vi "Set plot visibility.vi"(9 "Data In":T2, 10 "Timeline":T1, 11 "WaveformGraph in":T7) -> (3 "WaveformGraph out":T7)   [LabVIEW 2017, in "XGrapher.xctl"]
uses:
  XGrapher.xctl
  Typedefs/Xctrl-Waveform graph ref.ctl
  Data 1.ctl
  Typedefs/Xctrl-Data array.ctl
  Typedefs/Xcrtl-Data format definition.ctl
  Typedefs/Xctl-XY data type definition.ctl
  Typedefs/Xctrl-ROI type enum.ctl
  Typedefs/Xctrl-Timeline graph ref.ctl
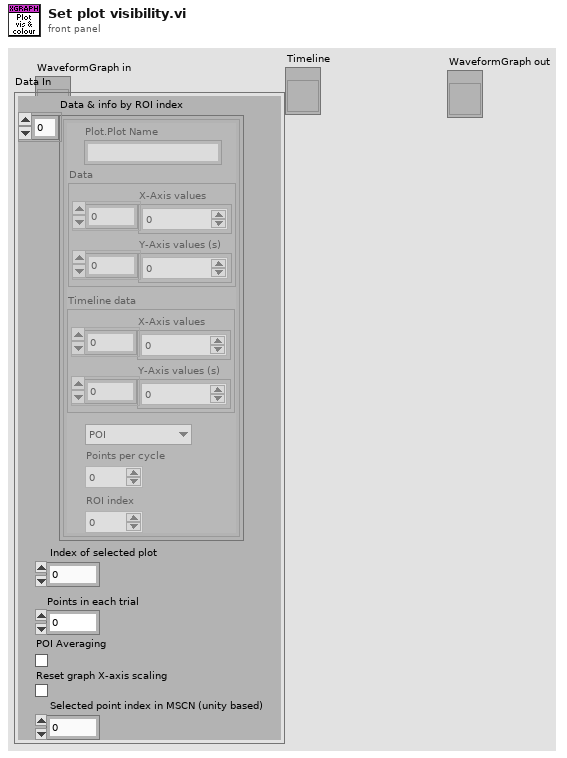
[diagram p1: front panel]
types:
  T1 = typedef "XGrapher.xctl/Xctrl-Timeline graph ref.ctl" = refnum<vi>
  T2 = typedef "XGrapher.xctl/Data 1.ctl" = cluster{"Data & info by ROI index":T3, "Index of selected plot":u16, "Points in each trial":i32, "POI Averaging":bool, "Reset graph X-axis scaling":bool, "Selected point index in MSCN (unity based)":u16}
  T3 = typedef "Xctrl-Data array.ctl" = T4[]
  T4 = typedef "XGrapher.xctl/Xcrtl-Data format definition.ctl" = cluster{"Plot.Plot Name":string, "Data":T5, "Timeline data":T5, "Type":T6, "Points per cycle":u16, "ROI index":u16}
  T5 = typedef "XGrapher.xctl/Xctl-XY data type definition.ctl" = cluster{"X-Axis values":sgl[], "Y-Axis values (s)":sgl[]}
  T6 = typedef "Xctrl-ROI type enum.ctl" = enum16{"POI", "Mini-scan", "Group"}
  T7 = typedef "XGrapher.xctl/Xctrl-Waveform graph ref.ctl" = refnum<vi>
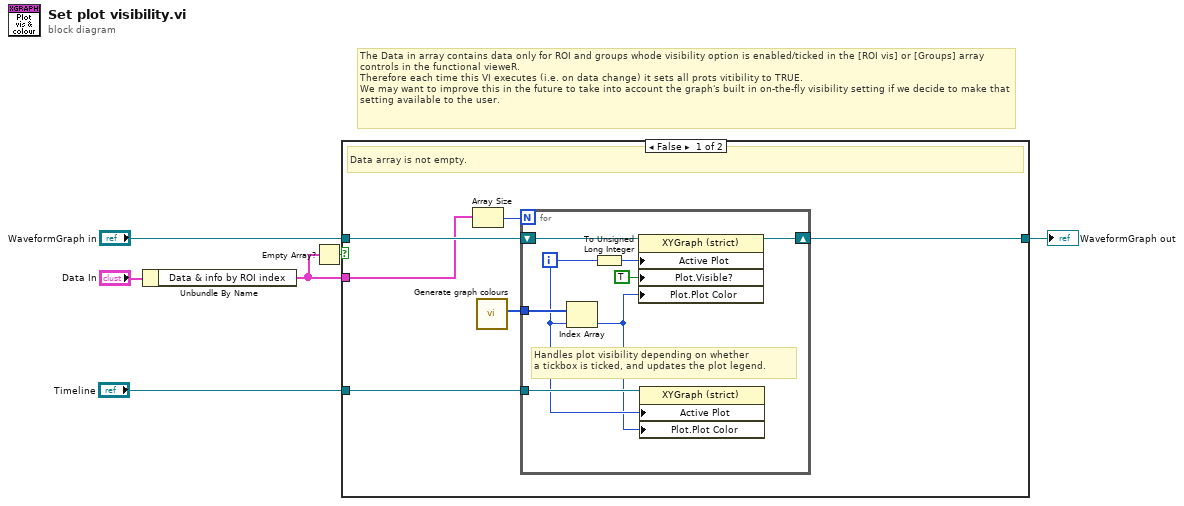
[diagram p0: block diagram]
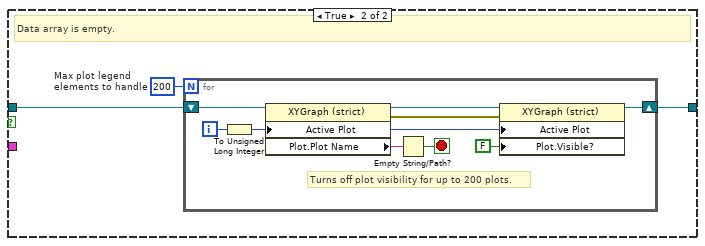
[diagram p2: hidden frame]
diagram:
  # "The Data in array contains data only for ROI and groups whode visibility option is enabled/ticked in the [ROI vis] or [Groups] array controls in the functional vieweR.\nTherefore each time this VI executes (i.e. on data change) it sets all prots vitibility to TRUE.\nWe may want to improve this in the future to take into account the graph's built in on-the-fly visibility setting if we decide to make that setting available to the user."
  n1 = Unbundle By Name("Data In") -> ("Data & info by ROI index"=w3:T3)
  n2 = Empty Array?(array=w3) -> (empty?=w2:bool)
  n3 = case shown="False" w2 {
    tunnel: "WaveformGraph in" -> [w12 w22]
    tunnel: [w11 w21] -> w5
    tunnel: w3 -> [w8 _]
    tunnel: "Timeline" -> [w7 _]
    frame False {
      # "Data array is not empty."
      n4 = Array Size(array=w8) -> (size(s)=w9:i32)
      n5 = call "Generate graph colours.vi"() -> ("Colours"=w10:u32[])  [unwired: 11 in]
      n6 = for {
        N: w9 -> [_]
        shift-right: [w19] -> w11
        shift-left: w12 -> [w20]
        tunnel: w10 -> [w16]
        tunnel: w7 -> [w15]
        i -> [w14]
        # "Handles plot visibility depending on whether\na tickbox is ticked, and updates the plot legend."
        n7 = Index Array(array=w16, index=w14) -> (element=w13:u32)
        n8 = To Unsigned Long Integer(number=w14) -> (unsigned 32bit integer=w18:u32)
        n9 = property on="Property Node" class="XYGraph (strict)"(reference=w20, "Active Plot"=w18, "Plot.Visible?"=TRUE ("Plot.Visible"), "Plot.Plot Color"=w13) -> (reference out=w19:T7)  [unwired: 1 in, 1 out]
        n10 = property on="Property Node" class="XYGraph (strict)"(reference=w15, "Active Plot"=w14, "Plot.Plot Color"=w13) -> ()  [unwired: 1 in, 2 out]
      }
    }
    frame True {
      w23 = 200  # Max plot legend elements to handle
      # "Data array is empty."
      n11 = for {
        N: w23 -> [_]
        shift-right: [w32] -> w21
        shift-left: w22 -> [w30]
        i -> [w25]
        stop <- w27 stop-if-true
        # "Turns off plot visibility for up to 200 plots."
        n12 = To Unsigned Long Integer(number=w25) -> (unsigned 32bit integer=w31:u32)
        n13 = property on="Property Node" class="XYGraph (strict)"(reference=w30, "Active Plot"=w31) -> (reference out=w29:T7, error out=w26:errorcluster, "Plot.Plot Name"=w28:string)  [unwired: 1 in]
        n14 = Empty String/Path?(string/path=w28) -> (empty?=w27:bool)
        n15 = property on="Property Node" class="XYGraph (strict)"(reference=w29, error in=w26, "Active Plot"=w31, "Plot.Visible?"=FALSE ("Plot.Visible")) -> (reference out=w32:T7)  [unwired: 1 out]
      }
    }
  }
  "WaveformGraph out" <- w5
